vi "readIRF.vi"(8 "Error In":errorcluster) -> (0 "Error Out":errorcluster, 2 "iRF out":dbl[](array[numeric]), 3 "iRF file path":path)   [LabVIEW 2020]
uses:
  <vilib>/Utility/file.llb/Read Delimited Spreadsheet (DBL).vi
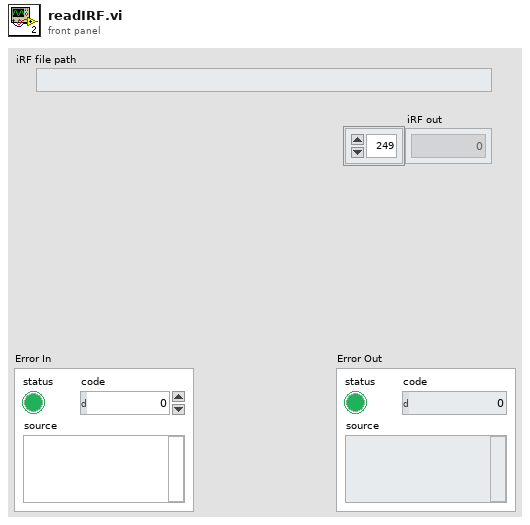
[diagram p1: front panel]
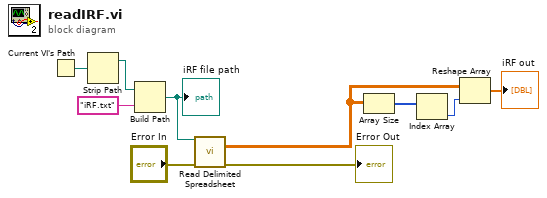
[diagram p0: block diagram]
diagram:
  n1 = Current VI's Path() -> (path=w10:path)
  n2 = Strip Path(path=w10) -> (stripped path=w9:path)  [unwired: 1 out]
  n3 = Build Path(base path=w9, name or relative path="iRF.txt") -> (appended path=w7:path)
  "iRF file path" <- w7
  n4 = call-poly <vilib>:"Read Delimited Spreadsheet.vi"("file path (dialog if empty)"=w7, "error in (no error)"="Error In") -> ("all rows"=w6:dbl[][], "error out"=→"Error Out":errorcluster)  [unwired: 8 in, 4 out]
  n5 = Array Size(array=w6) -> (size(s)=w5:i32[])
  n6 = Index Array(array=w5) -> (element=w4:i32)  [unwired: 1 in]
  n7 = Reshape Array(w6, w4) -> (→"iRF out":dbl[])
